vi "Cron Minutes.vi"(7 "Cron":refnum<class "Cron.lvclass">, 10 "Cron":T1) -> (2 "Cron Time":T1)   [LabVIEW 2013, in "openCron.lvlib" / "Cron.lvclass"]
uses:
  Cron.lvclass
  CronTime -- cluster.ctl
  Cron Interval -- enum.ctl
  Cron.lvclass/Cron.ctl
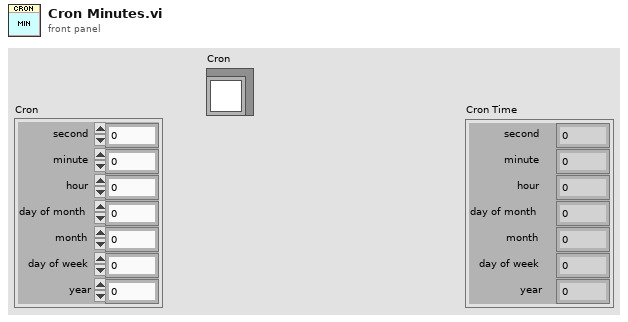
[diagram p1: front panel]
types:
  T1 = typedef "openCron.lvlib/Cron.lvclass/CronTime -- cluster.ctl" = cluster{"second":i32, "minute":i32, "hour":i32, "day of month":i32, "month":i32, "day of week":i32, "year":i32}
  T2 = typedef "openCron.lvlib/Cron.lvclass/Cron Interval -- enum.ctl" = enum16{"Seconds", "Minutes", "Hours", "Day of Month", "Month", "Day of Week", "Year"}
  T3 = typedef "openCron.lvlib/Cron.lvclass/Cron Interval -- cluster.ctl" = cluster{"Values":i32[], "All":bool, "Any":bool}
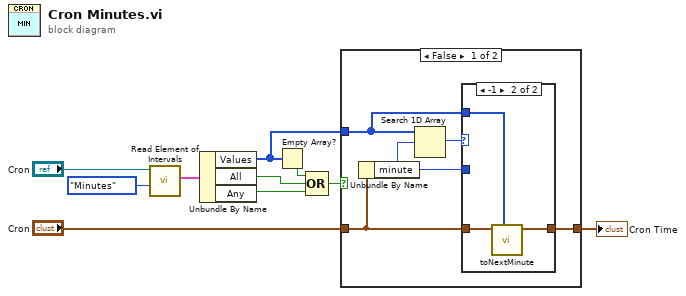
[diagram p0: block diagram]
diagram:
  n1 = call "Read Element of Intervals.vi"("Interval"=Cron_Interval_--_enum."Minutes", "Cron in"="Cron") -> ("Interval"=w6:T3)  [unwired: 7 in, 2 out]
  n2 = Unbundle By Name(w6) -> ("Values"=w1:i32[], "All"=w4:bool, "Any"=w5:bool)
  n3 = Empty Array?(array=w1) -> (empty?=w3:bool)
  n4 = Compound Arithmetic op=OR(w3, w4, w5) -> (w2:bool)
  n5 = case shown="False" w2 {
    tunnel: [w14 w20] -> w8
    tunnel: "Cron" -> [w15 w20]
    tunnel: w1 -> [w11 _]
    frame False {
      n6 = Unbundle By Name(w15) -> ("minute"=w13:i32)
      n7 = Search 1D Array(1D array=w11, element=w13) -> (index of element=w12:i32)  [unwired: 1 in]
      n8 = case shown="-1" w12 {
        tunnel: w15 -> [w16 w19]
        tunnel: [w16 w18] -> w14
        tunnel: w13 -> [_ _]
        tunnel: w11 -> [_ w17]
        frame 0, Default {
        }
        frame -1 {
          n9 = call "toNextMinute.vi"("Values"=w17, "Cron in"=w19) -> ("Cron out"=w18:T1)  [unwired: 9 in]
        }
      }
    }
    frame True {
    }
  }
  "Cron Time" <- w8
